vi "Workspace.CAN.TransportProtocol.Get.vi"(8 "error in (no error)":errorcluster, 10 "Path":string, 11 "NIVS.SysDef Ref":refnum<k24>) -> (0 "error out":errorcluster, 2 "Transport Protocol":T1, 3 "NIVS.SysDef Ref out":refnum<k24>)   [LabVIEW 2019, in "Diagnostics Workspace Shared.lvlib"]
uses:
  NationalInstruments.VeriStand.SystemStorage
  Addon/Addon Shared/Types/Transport.ctl
  NationalInstruments.VeriStand
  Addon/Addon Shared/SubVIs/Constants.vi
  Diagnostics Workspace Shared.lvlib
  Addon/Addon Shared/Diagnostics Addon Shared.lvlib
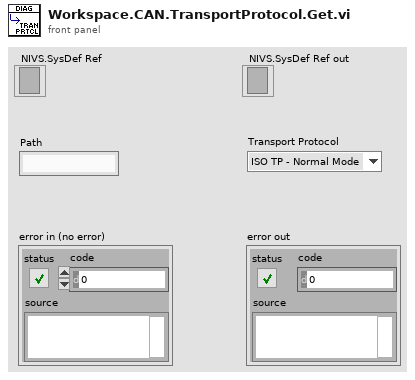
[diagram p1: front panel]
types:
  T1 = typedef "Diagnostics Addon Shared.lvlib/Transport.ctl" = enum16{"ISO TP - Normal Mode", "ISO TP - Mixed Mode", "VW TP 2.0", "Diagnostics on IP", "ISO TP LIN"}
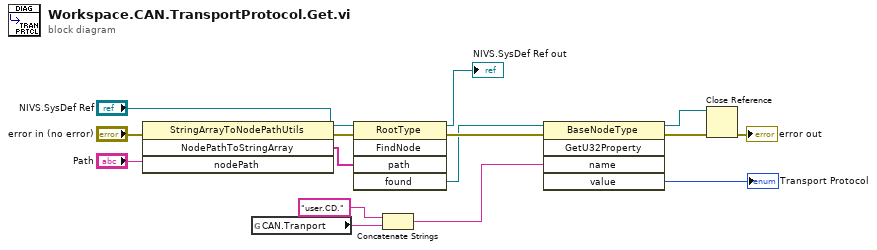
[diagram p0: block diagram]
diagram:
  n1 = invoke class="StringArrayToNodePathUtils" method="NodePathToStringArray"(error in="error in (no error)", "nodePath"="Path") -> (error out=w10:errorcluster, "NodePathToStringArray"=w12:string[])  [unwired: 2 in, 2 out]
  n2 = global read "Constants.vi" "CAN.Tranport"() -> (w15:string)
  n3 = invoke class="RootType" method="FindNode"(reference="NIVS.SysDef Ref", error in=w10, "path"=w12) -> (reference out=→"NIVS.SysDef Ref out":refnum<k24>, error out=w14:errorcluster, "found"=w7:refnum<k24>)  [unwired: 2 in, 2 out]
  n4 = Concatenate Strings("user.CD." ("string"), w15) -> (w5:string)
  n5 = invoke class="BaseNodeType" method="GetU32Property"(reference=w7, error in=w14, "name"=w5) -> (reference out=w3:refnum<k24>, error out=w4:errorcluster, "value"=→"Transport Protocol":u32)  [unwired: 2 in, 2 out]
  n6 = Close Reference(reference=w3, error in (no error)=w4) -> (error out=→"error out":errorcluster)
